vi "项操作.vi"(8 "error in (no error)":errorcluster caption="错误输入（无错误）", 9 "Cell Position":T1, 10 "MCListbox引用句柄":refnum<vi>, 11 "LNK 输入":refnum<class "Menu.lvclass">) -> (0 "error out":errorcluster caption="错误输出", 3 "LNK 输出":refnum<class "Menu.lvclass">)   [LabVIEW 2016, in "Menu.lvclass"]
uses:
  Menu.lvclass
  <vilib>/Utility/miscctls.llb/LVRowAndColumnTypeDef.ctl
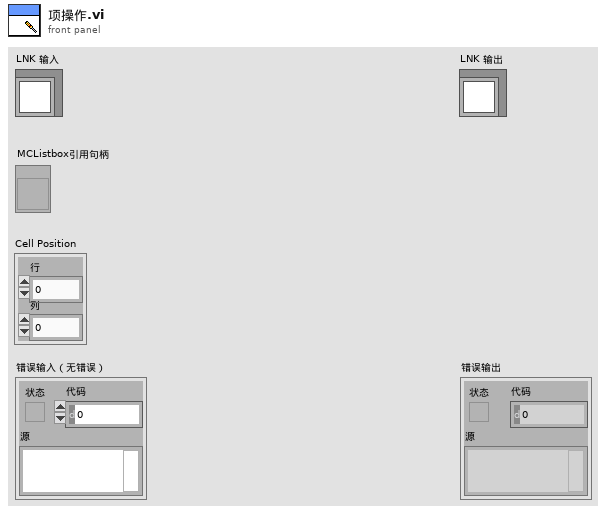
[diagram p1: front panel]
types:
  T1 = typedef "LVRowAndColumnTypeDef.ctl" = cluster{"Row":i32, "Column":i32}
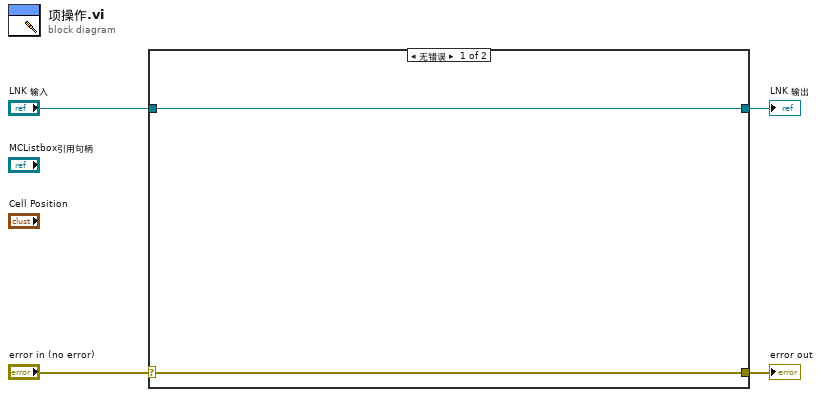
[diagram p0: block diagram]
diagram:
  n1 = case shown="无错误" "error in (no error)" {
    selector: "error in (no error)" -> [w5 w8]
    tunnel: [w5 w8] -> w3
    tunnel: [w6 w7] -> w1
    tunnel: "LNK 输入" -> [w6 w7]
    frame No Error {
    }
    frame Error {
    }
  }
  "error out" <- w3
  "LNK 输出" <- w1
